vi "Test My Cloneable Module API.vi"() -> ()   [LabVIEW 2020]
doc: "My Module API Tester.\n_____\nBased on Delacor QMH Project Template 5.1.0.87."
uses:
  My Cloneable Module.lvlib
panel:
  in  "FP Color":u32(colorbox)
  in  "Change FP Color":bool
  in  "wait for reply":bool=TRUE
  in  "Run as Singleton?":bool
  in  "Show Block Diagram":bool
  in  "Refresh Modules":bool
  in  "X":dbl=1.0
  out "Reply Payload":dbl
  out "Active Modules":string[](array[string])
  in  "Stop Module":bool
  in  "Select Module":i32(ring)=-1 caption="Select Module\nTo send Request to" items=["All"=-1]
  in  "Run New Module":bool
  out "Do Something Count":i32
  in  "Test Do Something Else and Wait for Reply":bool
  in  "Hide Module Panel":bool
  in  "Show Module Panel":bool
  in  "Test Do Something Else":bool
  in  "Test Do Something":bool
  out "Status":string
  # "This VI tests the API for the Module."
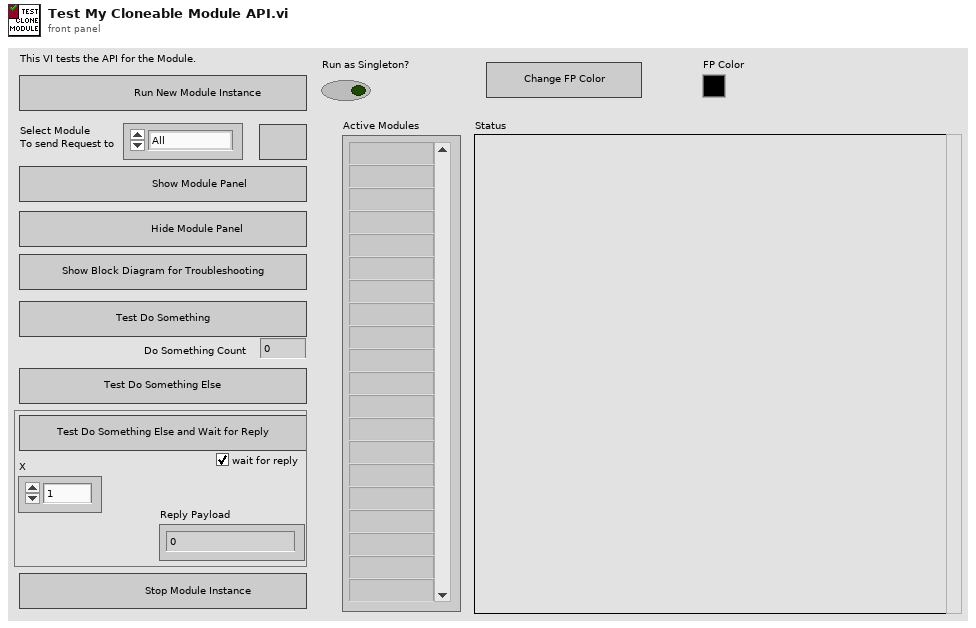
[diagram p1: front panel]
types:
  T1 = typedef "My Cloneable Module.lvlib/Broadcast Events--cluster.ctl" = cluster{"Module Did Init":refnum<user-event>, "Status Updated":refnum<user-event>, "Error Reported":refnum<user-event>, "Did Something":refnum<user-event>, "Module Did Stop":refnum<user-event>, "Update Module Execution Status":refnum<user-event>}
  T2 = typedef "My Cloneable Module.lvlib/Do Something Else and Wait (Reply Payload)--cluster.ctl" = cluster{"Value":dbl, "error":errorcluster}
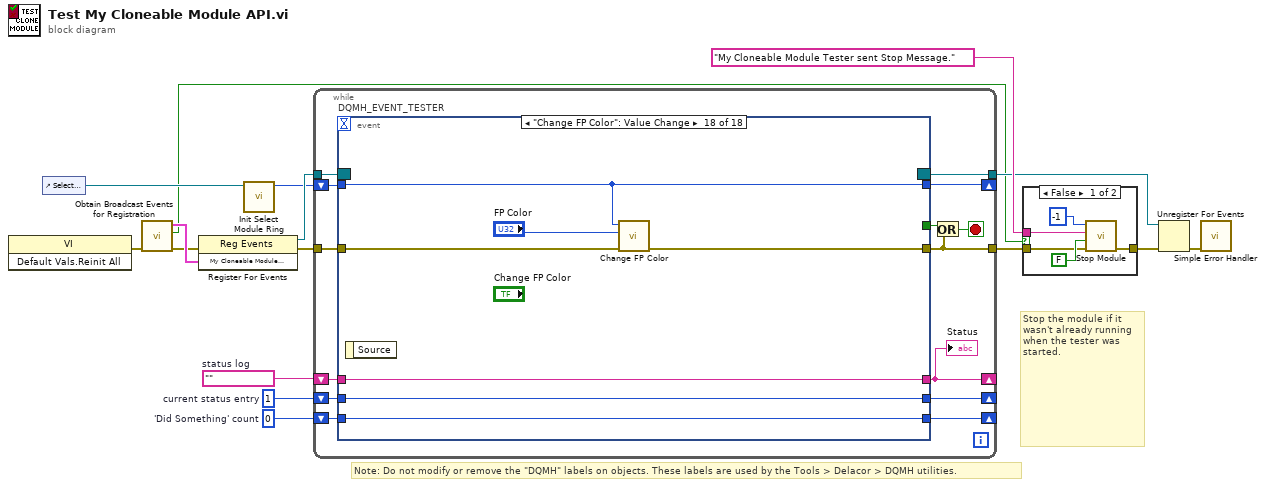
[diagram p0: block diagram]
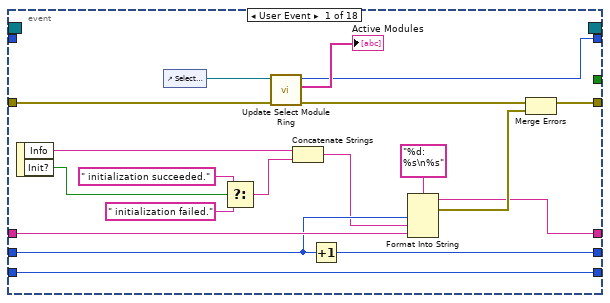
[diagram p3: hidden frame]
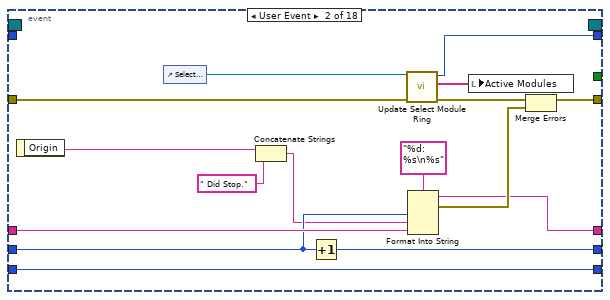
[diagram p4: hidden frame]
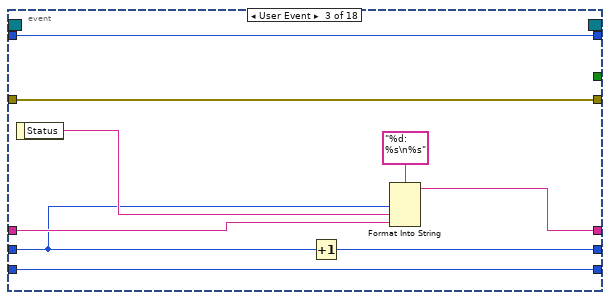
[diagram p5: hidden frame]
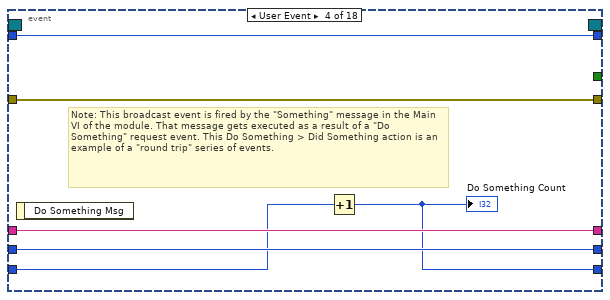
[diagram p6: hidden frame]
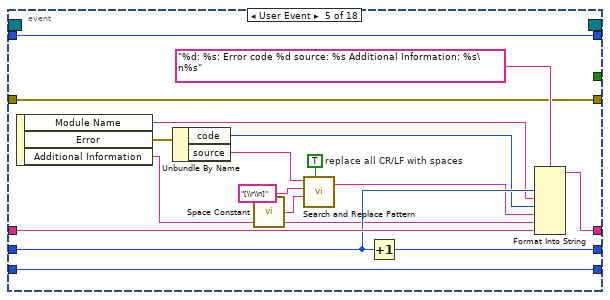
[diagram p7: hidden frame]
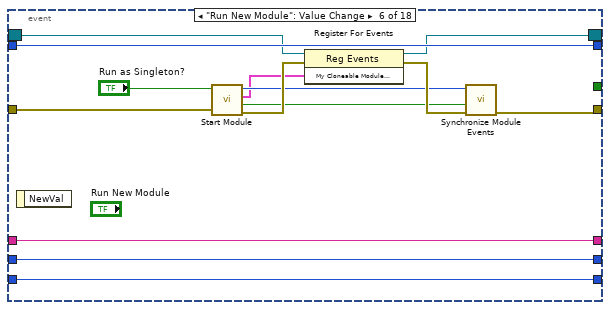
[diagram p8: hidden frame]
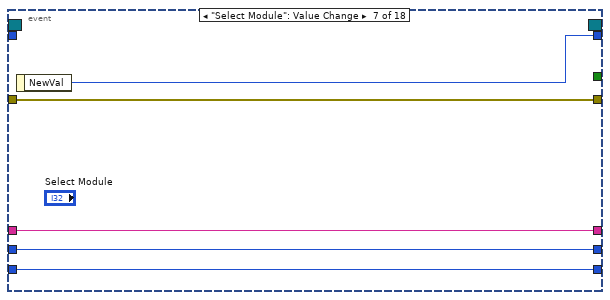
[diagram p9: hidden frame]
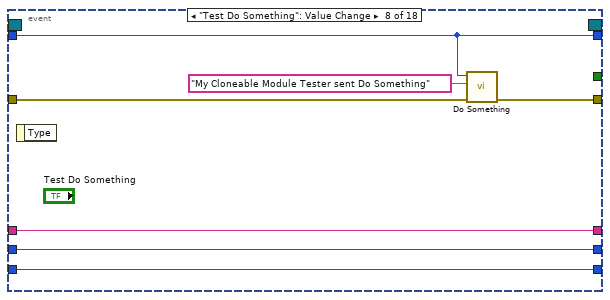
[diagram p10: hidden frame]
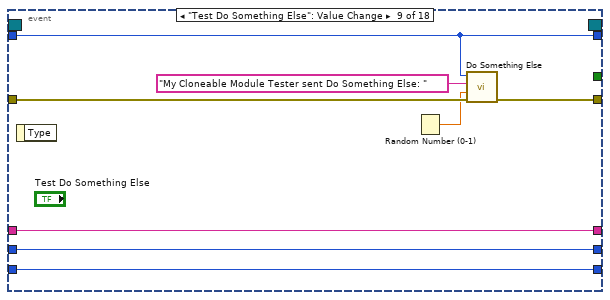
[diagram p11: hidden frame]
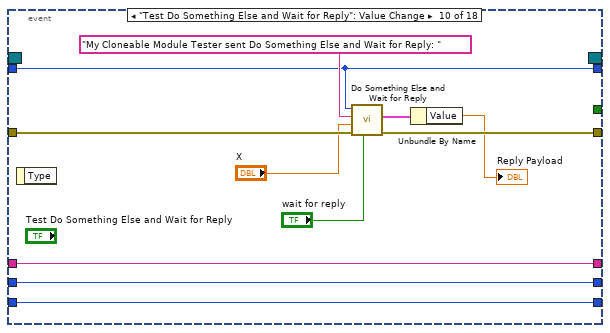
[diagram p12: hidden frame]
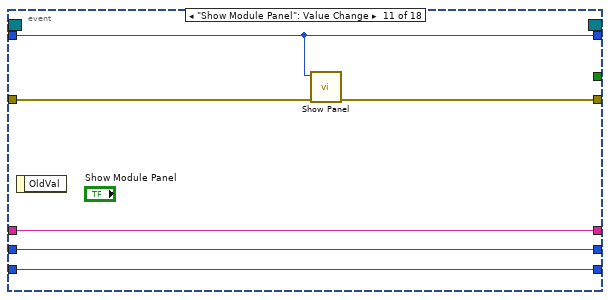
[diagram p13: hidden frame]
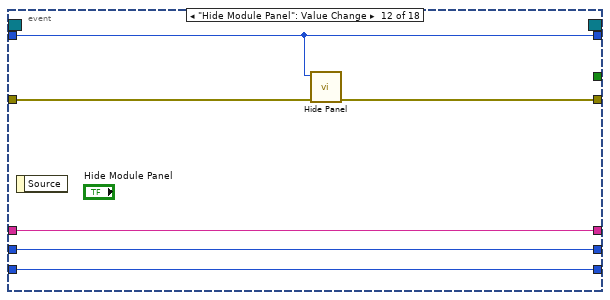
[diagram p14: hidden frame]
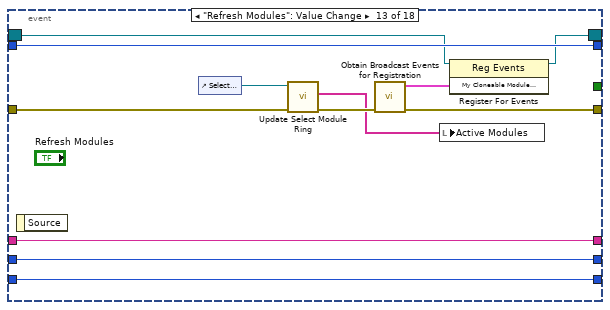
[diagram p15: hidden frame]
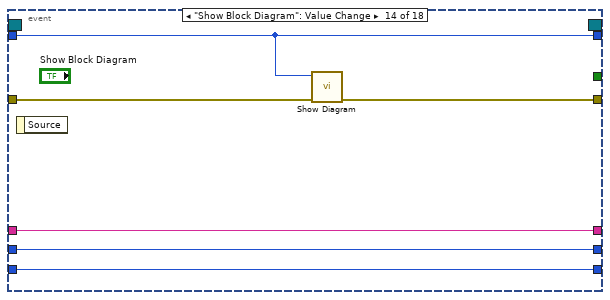
[diagram p16: hidden frame]
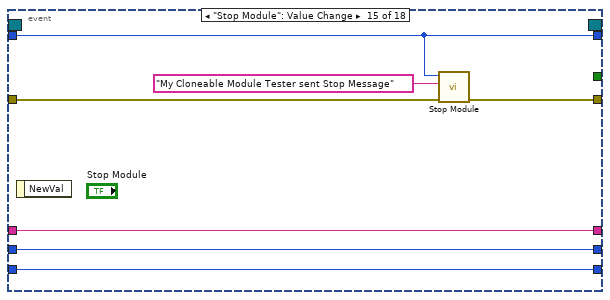
[diagram p17: hidden frame]
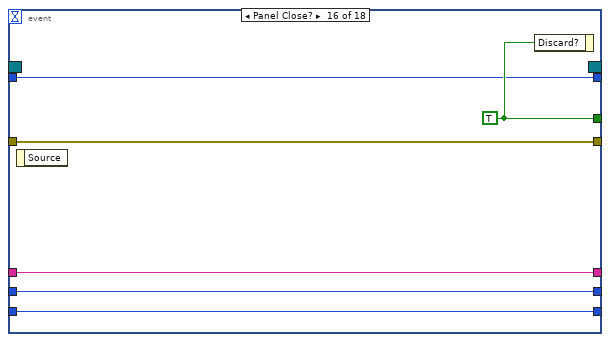
[diagram p18: hidden frame]
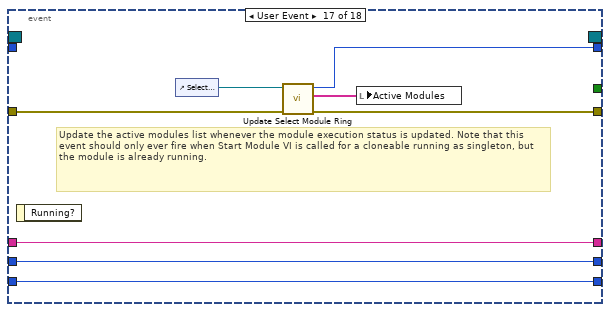
[diagram p19: hidden frame]
diagram:
  w12 = 0  # 'Did Something' count
  w13 = 1  # current status entry
  w14 = ""  # status log
  # "Stop the module if it wasn't already running when the tester was started."
  # "Note: Do not modify or remove the \"DQMH\" labels on objects. These labels are used by the Tools > Delacor > DQMH utilities."
  n1 = invoke class="VI" method="Default Vals.Reinit All"() -> (error out=w5:errorcluster)  [unwired: 3 in, 2 out]
  n2 = control-ref of="Select Module"() -> (w10:refnum<vi>)
  n3 = call "Obtain Broadcast Events for Registration.vi"("error in (no error)"=w5) -> ("error out"=w4:errorcluster, "Already running?"=w3:bool, "My Cloneable Module Broadcast Events"=w9:T1)  [unwired: 8 in]
  n4 = register-events(error in=w4, w9) -> (reference out=w16:refnum<event-registration>, error out=w8:errorcluster)  [unwired: 1 in]
  n5 = call "Init Select Module Ring.vi"("Select Module Ring Ref"=w10) -> ("Value for All Modules"=w11:i32)  [unwired: 8 in, 2 out]
  n6 = while {
    tunnel: w16 -> [w30]
    tunnel: [w17] -> w2
    tunnel: w8 -> [w28]
    shift-right: [w24] -> _
    shift-left: w14 -> [w26]
    shift-right: [w25] -> _
    shift-left: w13 -> [w27]
    shift-right: [w22] -> _
    shift-left: w12 -> [w23]
    shift-right: [w19] -> _
    shift-left: w11 -> [w20]
    tunnel: [w18] -> w6
    stop <- w21 stop-if-true
    n7 = event "DQMH_EVENT_TESTER" shown="[17] \"Change FP Color\": Value Change" {
      selector: w30 -> [_ _ _ _ _ w104 _ _ _ _ _ _ w160 _ _ _ _ _]
      dyn-events: [_ _ _ _ _ w103 _ _ _ _ _ _ w159 _ _ _ _ _] -> w18
      timeout: _ -> [_ _ _ _ _ _ _ _ _ _ _ _ _ _ _ _ _ _]
      tunnel: [_ _ _ _ _ _ _ _ _ _ _ _ _ _ _ w185 _ _] -> w29
      tunnel: [w38 w56 w74 w80 w86 w102 w116 w122 w130 w142 w147 w153 w156 w168 w174 w184 w188 w196] -> w17
      tunnel: w28 -> [w40 w58 w74 w80 w86 w105 w116 w123 w131 w134 w148 w154 w161 w172 w175 w184 w189 w200]
      tunnel: w27 -> [w46 w62 w66 w78 w92 w108 w114 w119 w126 w139 w145 w151 w165 w170 w178 w182 w192 w198]
      tunnel: w26 -> [w47 w63 w70 w79 w94 w109 w115 w120 w127 w140 w146 w152 w166 w171 w179 w183 w193 w199]
      tunnel: [w44 w60 w71 w79 w89 w109 w115 w120 w127 w140 w146 w152 w166 w171 w179 w183 w193 w199] -> w24
      tunnel: [w45 w61 w73 w78 w95 w108 w114 w119 w126 w139 w145 w151 w165 w170 w178 w182 w192 w198] -> w25
      tunnel: w23 -> [w41 w59 w69 w77 w97 w107 w113 w118 w125 w138 w144 w150 w164 w169 w177 w181 w191 w197]
      tunnel: [w41 w59 w69 w76 w97 w107 w113 w118 w125 w138 w144 w150 w164 w169 w177 w181 w191 w197] -> w22
      tunnel: w20 -> [_ _ w67 w75 w96 w106 _ w117 w124 w137 w143 w149 w163 w167 w176 w180 _ w195]
      tunnel: [w35 w53 w67 w75 w96 w106 w112 w117 w124 w137 w143 w149 w163 w167 w176 w180 w187 w195] -> w19
      event User Event {
        n8 = event-data() -> ("Info"=w43:string, "Init?"=w32:bool)  [unwired: 1 in]
        n9 = control-ref of="Select Module"() -> (w37:refnum<vi>)
        n10 = Select(t=" initialization succeeded.", s=w32, f=" initialization failed.") -> (s? t:f=w31:string)
        n11 = call "Update Select Module Ring.vi"("error in (no error)"=w40, "Select Module Ring Ref"=w37) -> ("error out"=w39:errorcluster, "Active Modules (Array)"=→"Active Modules":string[], "New Module Ring Value"=w35:i32)  [unwired: 7 in]
        n12 = Concatenate Strings(w43, w31) -> (w42:string)
        n13 = Increment(x=w46) -> (x+1=w45:i32)
        n14 = Format Into String(format string="%d: %s\n%s", w46, w42, w47) -> (resulting string=w44:string, error out=w49:errorcluster)  [unwired: 2 in]
        n15 = Merge Errors(w39, w49) -> (w38:errorcluster)
      }
      event User Event {
        n16 = event-data() -> ("Origin"=w51:string)  [unwired: 1 in]
        n17 = control-ref of="Select Module"() -> (w55:refnum<vi>)
        n18 = Concatenate Strings(w51, " Did Stop.") -> (w50:string)
        n19 = Increment(x=w62) -> (x+1=w61:i32)
        n20 = call "Update Select Module Ring.vi"("error in (no error)"=w58, "Select Module Ring Ref"=w55) -> ("error out"=w57:errorcluster, "Active Modules (Array)"=w54:string[], "New Module Ring Value"=w53:i32)  [unwired: 7 in]
        n21 = Format Into String(format string="%d: %s\n%s", w62, w50, w63) -> (resulting string=w60:string, error out=w65:errorcluster)  [unwired: 2 in]
        n22 = local write "Active Modules"(w54) -> ()
        n23 = Merge Errors(w57, w65) -> (w56:errorcluster)
      }
      event User Event {
        n24 = event-data() -> ("Status"=w68:string)  [unwired: 1 in]
        n25 = Increment(x=w66) -> (x+1=w73:i32)
        n26 = Format Into String(format string="%d: %s\n%s", w66, w68, w70) -> (resulting string=w71:string)  [unwired: 2 in, 1 out]
      }
      event User Event {
        # "Note: This broadcast event is fired by the \"Something\" message in the Main VI of the module. That message gets executed as a result of a \"Do Something\" request event. This Do Something > Did Something action is an example of a \"round trip\" series of events."
        n27 = event-data() -> ()  [unwired: 1 in, 1 out]
        n28 = Increment(x=w77) -> (x+1=w76:i32)
        "Do Something Count" <- w76
      }
      event User Event {
        w90 = TRUE  # replace all CR/LF with spaces
        n29 = event-data() -> ("Module Name"=w84:string, "Error"=w83:errorcluster, "Additional Information"=w81:string)  [unwired: 1 in]
        n30 = Unbundle By Name(w83) -> ("code"=w85:i32, "source"=w87:string)
        n31 = call <vilib>:"Space Constant.vi"() -> ("String"=w91:string)
        n32 = call <vilib>:"Search and Replace Pattern.vi"("string"=w87, "regular expression (\"\")"="[\\r\\n]" ("regular expression (\"\")"), "replace string (\"\")"=w91, "replace all? (F)"=w90) -> ("result string"=w88:string)  [unwired: 1 in, 1 out]
        n33 = Increment(x=w92) -> (x+1=w95:i32)
        n34 = Format Into String(format string="%d: %s: Error code %d source: %s Additional Information: %s\n%s", w92, w84, w85, w88, w81, w94) -> (resulting string=w89:string)  [unwired: 2 in, 1 out]
      }
      event "Run New Module": Value Change {
        n35 = event-data() -> ()  [unwired: 1 in, 1 out]
        n36 = call "Start Module.vi"("error in"=w105, "Run as Singleton? (F)"="Run as Singleton?") -> ("error out"=w110:errorcluster, "Wait for Event Sync?"=w100:bool, "My Cloneable Module Broadcast Events"=w99:T1, "Module ID"=w101:i32)  [unwired: 6 in]
        n37 = register-events(reference=w104, error in=w110, w99) -> (reference out=w103:refnum<event-registration>, error out=w111:errorcluster)
        n38 = call "Synchronize Module Events.vi"("error in"=w111, "Wait for Event Sync?"=w100, "Module ID in"=w101) -> ("error out"=w102:errorcluster)  [unwired: 7 in, 1 out]
      }
      event "Select Module": Value Change {
        n39 = event-data() -> ("NewVal"=w112:i32)  [unwired: 1 in]
      }
      event "Test Do Something": Value Change {
        n40 = event-data() -> ()  [unwired: 1 in, 1 out]
        n41 = call "Do Something.vi"("error in (no error)"=w123, "Do Something Message"="My Cloneable Module Tester sent Do Something", "Module ID"=w117) -> ("error out"=w122:errorcluster)  [unwired: 8 in]
      }
      event "Test Do Something Else": Value Change {
        n42 = event-data() -> ()  [unwired: 1 in, 1 out]
        n43 = Random Number (0-1)() -> (number: 0 to 1=w128:dbl)
        n44 = call "Do Something Else.vi"("error in (no error)"=w131, "X"=w128, "Do Something else Message"="My Cloneable Module Tester sent Do Something Else: " ("Do Something Message"), "Module ID"=w124) -> ("error out"=w130:errorcluster)  [unwired: 7 in]
      }
      event "Test Do Something Else and Wait for Reply": Value Change {
        n45 = event-data() -> ()  [unwired: 1 in, 1 out]
        n46 = call "Do Something Else and Wait for Reply.vi"("wait for reply (T)"="wait for reply", "error in (no error)"=w134, "X"="X", "Do Something Else Message"="My Cloneable Module Tester sent Do Something Else and Wait for Reply: " ("Do Something Message"), "Module ID"=w137) -> ("error out"=w142:errorcluster, "Reply Payload"=w136:T2)  [unwired: 4 in, 1 out]
        n47 = Unbundle By Name(w136) -> ("Value"=→"Reply Payload":dbl)
      }
      event "Show Module Panel": Value Change {
        n48 = event-data() -> ()  [unwired: 1 in, 1 out]
        n49 = call "Show Panel.vi"("error in (no error)"=w148, "Module ID"=w143) -> ("error out"=w147:errorcluster)  [unwired: 9 in]
      }
      event "Hide Module Panel": Value Change {
        n50 = event-data() -> ()  [unwired: 1 in, 1 out]
        n51 = call "Hide Panel.vi"("error in (no error)"=w154, "Module ID"=w149) -> ("error out"=w153:errorcluster)  [unwired: 9 in]
      }
      event "Refresh Modules": Value Change {
        n52 = event-data() -> ()  [unwired: 1 in, 1 out]
        n53 = control-ref of="Select Module"() -> (w162:refnum<vi>)
        n54 = call "Update Select Module Ring.vi"("error in (no error)"=w161, "Select Module Ring Ref"=w162) -> ("error out"=w157:errorcluster, "Active Modules (Array)"=w155:string[])  [unwired: 7 in, 1 out]
        n55 = call "Obtain Broadcast Events for Registration.vi"("error in (no error)"=w157) -> ("error out"=w156:errorcluster, "My Cloneable Module Broadcast Events"=w158:T1)  [unwired: 8 in, 1 out]
        n56 = local write "Active Modules"(w155) -> ()
        n57 = register-events(reference=w160, w158) -> (reference out=w159:refnum<event-registration>)  [unwired: 1 in, 1 out]
      }
      event "Show Block Diagram": Value Change {
        n58 = event-data() -> ()  [unwired: 1 in, 1 out]
        n59 = call "Show Diagram.vi"("error in (no error)"=w172, "Module ID"=w167) -> ("error out"=w168:errorcluster)  [unwired: 9 in]
      }
      event "Stop Module": Value Change {
        n60 = event-data() -> ()  [unwired: 1 in, 1 out]
        n61 = call "Stop Module.vi"("error in (no error)"=w175, "Origin"="My Cloneable Module Tester sent Stop Message", "Module ID"=w176) -> ("error out"=w174:errorcluster)  [unwired: 8 in]
      }
      event Panel Close? {
        w185 = TRUE ("Discard?")
        n62 = event-data() -> ()  [unwired: 1 in, 1 out]
        n63 = event-data("Discard?"=w185) -> ()  [unwired: 1 in, 1 out]
      }
      event User Event {
        # "Update the active modules list whenever the module execution status is updated. Note that this event should only ever fire when Start Module VI is called for a cloneable running as singleton, but the module is already running."
        n64 = event-data() -> ()  [unwired: 1 in, 1 out]
        n65 = control-ref of="Select Module"() -> (w190:refnum<vi>)
        n66 = call "Update Select Module Ring.vi"("error in (no error)"=w189, "Select Module Ring Ref"=w190) -> ("error out"=w188:errorcluster, "Active Modules (Array)"=w186:string[], "New Module Ring Value"=w187:i32)  [unwired: 7 in]
        n67 = local write "Active Modules"(w186) -> ()
      }
      event "Change FP Color": Value Change {
        n68 = event-data() -> ()  [unwired: 1 in, 1 out]
        n69 = call "Change FP Color.vi"("error in"=w200, "FP Color"="FP Color", "Module ID"=w195) -> ("error out"=w196:errorcluster)  [unwired: 8 in]
      }
    }
    "Status" <- w24
    n70 = Or(x=w29, y=w17) -> (x .or. y?=w21:bool)
  }
  n71 = case shown="False" w3 {
    tunnel: [w205 w206] -> w15
    tunnel: "My Cloneable Module Tester sent Stop Message." ("Origin") -> [w204 _]
    tunnel: w2 -> [w201 w206]
    frame False {
      n72 = call "Stop Module.vi"("error in (no error)"=w201, "Wait for Module to stop? (F)"=FALSE ("Wait for Module to stop?"), "Origin"=w204, "Module ID"=-1 ("Stop all")) -> ("error out"=w205:errorcluster)  [unwired: 7 in]
    }
    frame True {
    }
  }
  n73 = Unregister For Events(event registration refnum=w6, error in=w15) -> (error out=w1:errorcluster)
  n74 = call <vilib>:"Simple Error Handler.vi"("error in (no error)"=w1) -> ()  [unwired: 4 in, 5 out]
